vi "ConfigArbWfrmSRat.vi"(8 "error in (no error)":errorcluster, 11 "ClassIn":refnum<class "Keysight335XX.lvclass">) -> (0 "error out":errorcluster, 3 "ClassOut":refnum<class "Keysight335XX.lvclass">)   [LabVIEW 2014, in "FGenPlugins.lvlib" / "Keysight335XX.lvclass"]
uses:
  Keysight335XX.lvclass
  <instrlib>/Agilent 3352X Series/Agilent 3352X Series.lvlib
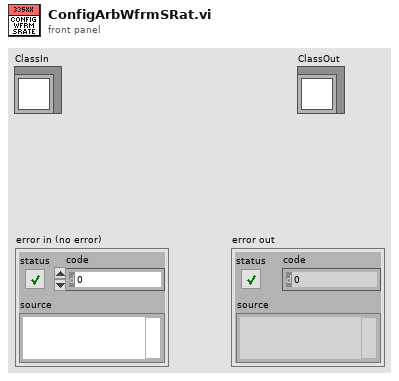
[diagram p1: front panel]
types:
  T1 = typedef "NISTFGenPlugins.lvlib/NISTFGenPluginsBase.lvclass/ArbWfrmParams.ctl" = cluster{"sWfrmHandle":string, "iSize":i32, "dData":dbl[], "dGain":dbl, "dOffset":dbl, "dSampleRate":dbl}
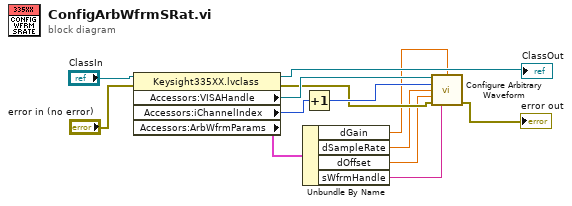
[diagram p0: block diagram]
diagram:
  n1 = property class="Keysight335XX.lvclass"(reference="ClassIn", error in="error in (no error)") -> (reference out=→"ClassOut":refnum<class "Keysight335XX.lvclass">, error out=w9:errorcluster, "Accessors:VISAHandle"=w13:refnum<visa-resource-name>, "Accessors:iChannelIndex"=w12:i32, "Accessors:ArbWfrmParams"=w10:T1)
  n2 = Unbundle By Name(w10) -> ("dGain"=w4:dbl, "dSampleRate"=w3:dbl, "dOffset"=w2:dbl, "sWfrmHandle"=w1:string)
  n3 = Increment(x=w12) -> (x+1=w11:i32)
  n4 = call <instrlib>:"Configure Arbitrary Waveform.vi"("VISA resource name"=w13, "Amplitude (0.1 Vpp)"=w4, "Channel (1: 1)"=w11, "Sample Rate (40000 Sa/s)"=w3, "Offset (0 V)"=w2, "error in (no error)"=w9, "Arbitrary Waveform (ARB1)"=w1) -> ("error out"=→"error out":errorcluster)  [unwired: 3 in, 5 out]
